vi "update_sampling_mode.vi"(8 "error in (no error)":errorcluster, 11 "GenericWriteSignals in":refnum<class "GenericSignalWriter.lvclass">) -> (0 "error out":errorcluster, 3 "GenericWriteSignals out":refnum<class "GenericSignalWriter.lvclass">)   [LabVIEW 2010, in "GenericSignalWriter.lvclass"]
uses:
  GenericSignalWriter.lvclass
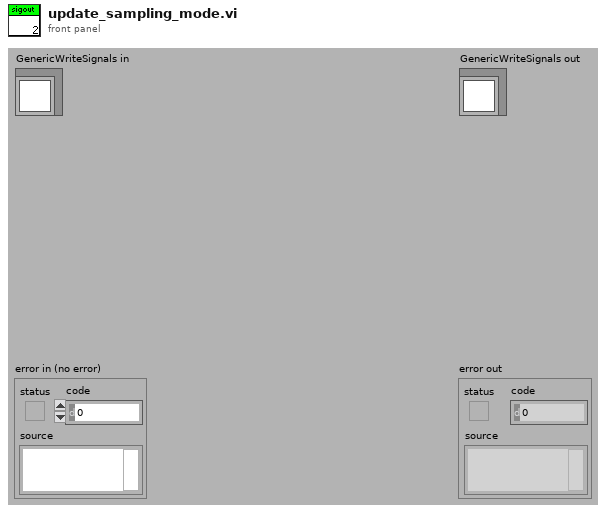
[diagram p1: front panel]
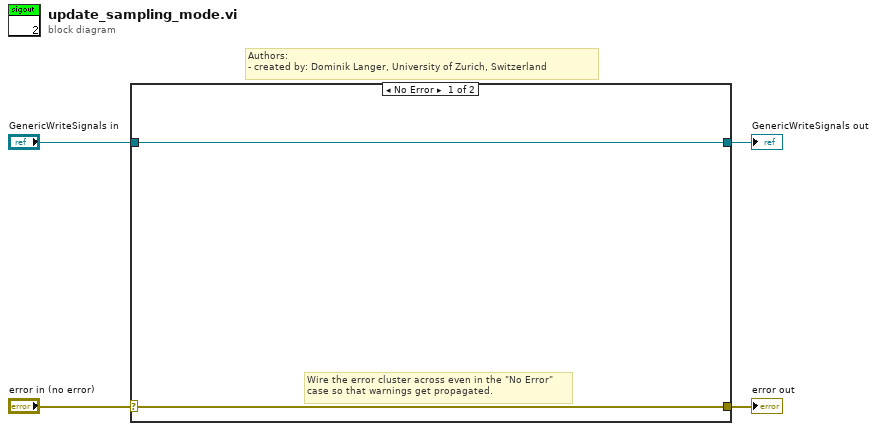
[diagram p0: block diagram]
diagram:
  # "Authors: \n- created by: Dominik Langer, University of Zurich, Switzerland"
  n1 = case shown="No Error" "error in (no error)" {
    selector: "error in (no error)" -> [w5 w8]
    tunnel: [w5 w8] -> w3
    tunnel: [w6 w7] -> w1
    tunnel: "GenericWriteSignals in" -> [w6 w7]
    frame No Error {
      # "Wire the error cluster across even in the \"No Error\"\ncase so that warnings get propagated."
    }
    frame Error {
    }
  }
  "error out" <- w3
  "GenericWriteSignals out" <- w1
